vi "PCAN_ERROR_Description.vi"(3 "error":T1 items=["CAN_ERR_OK"=0, "CAN_ERR_XMTFULL"=1, "CAN_ERR_OVERRUN"=2, "CAN_ERR_BUSLIGHT"=4, "CAN_ERR_BUSHEAVY"=8, "CAN_ERR_BUSOFF"=16, "CAN_ERR_QRCVEMPTY"=32, "CAN_ERR_QOVERRUN"=64, "CAN_ERR_QXMTFULL"=128, "CAN_ERR_REGTEST"=256, "CAN_ERR_NOVXD"=512, "CAN_ERR_HWINUSE"=1024, "CAN_ERR_NETINUSE"=2048, "CAN_ERR_ILLHW"=5120, "CAN_ERR_ILLNET"=6144, "CAN_ERR_ILLCLINET"=7168, "CAN_ERR_RESOURCE"=8192, "CAN_ERR_ILLPARAMTYPE"=16384, "CAN_ERR_ILLPARAMVAL"=32768, "CAN_ERR_UNKNOWN"=65536]) -> (1 "Error Description":string)   [LabVIEW 2010]
uses:
  PCAN_ERROR.ctl
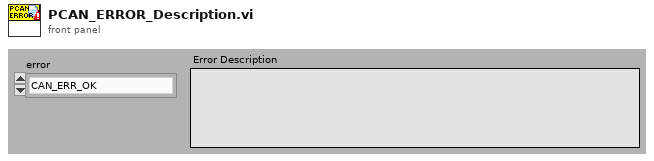
[diagram p1: front panel]
types:
  T1 = typedef "PCAN_ERROR.ctl" = i32
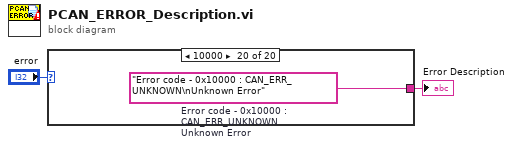
[diagram p0: block diagram]
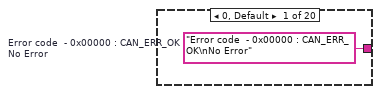
[diagram p2: hidden frame]
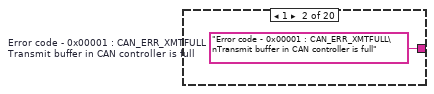
[diagram p3: hidden frame]
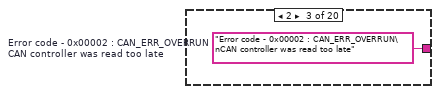
[diagram p4: hidden frame]
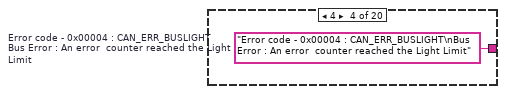
[diagram p5: hidden frame]
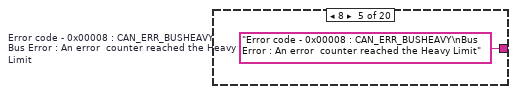
[diagram p6: hidden frame]
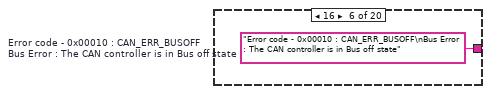
[diagram p7: hidden frame]
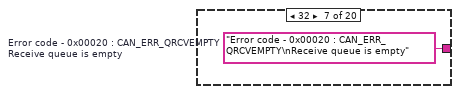
[diagram p8: hidden frame]
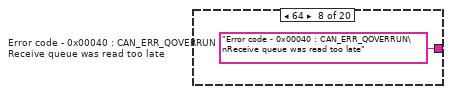
[diagram p9: hidden frame]
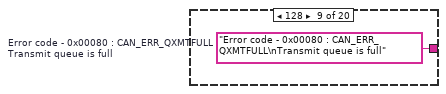
[diagram p10: hidden frame]
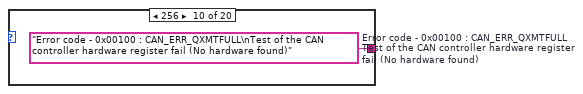
[diagram p11: hidden frame]
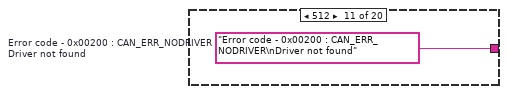
[diagram p12: hidden frame]
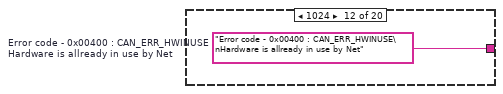
[diagram p13: hidden frame]
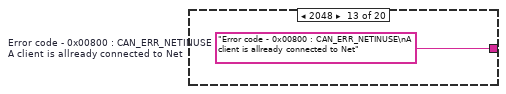
[diagram p14: hidden frame]
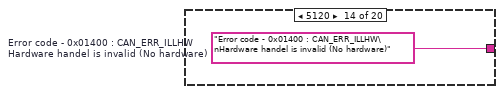
[diagram p15: hidden frame]
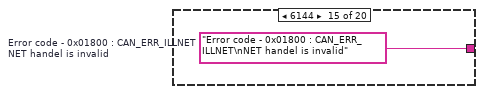
[diagram p16: hidden frame]
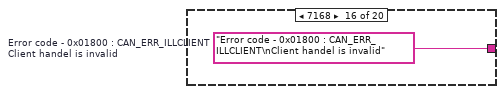
[diagram p17: hidden frame]
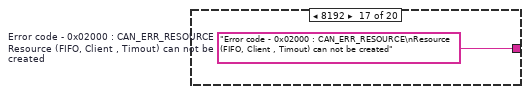
[diagram p18: hidden frame]
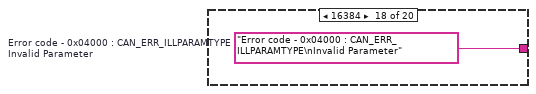
[diagram p19: hidden frame]
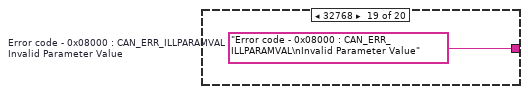
[diagram p20: hidden frame]
diagram:
  n1 = case shown="10000" "error" {
    tunnel: [w3 w4 w5 w6 w7 w8 w9 w10 w11 w12 w13 w14 w15 w16 w17 w18 w19 w20 w21 w22] -> w1
    frame 0, Default {
      w3 = "Error code  - 0x00000 : CAN_ERR_OK\nNo Error"  # Error code  - 0x00000 : CAN_ERR_OK No Error
    }
    frame 1 {
      w4 = "Error code - 0x00001 : CAN_ERR_XMTFULL\nTransmit buffer in CAN controller is full"  # Error code - 0x00001 : CAN_ERR_XMTFULL Transmit buffer in CAN controller is full
    }
    frame 2 {
      w5 = "Error code - 0x00002 : CAN_ERR_OVERRUN\nCAN controller was read too late"  # Error code - 0x00002 : CAN_ERR_OVERRUN CAN controller was read too late
    }
    frame 4 {
      w6 = "Error code - 0x00004 : CAN_ERR_BUSLIGHT\nBus Error : An error  counter reached the Light Limit"  # Error code - 0x00004 : CAN_ERR_BUSLIGHT Bus Error : An error  counter reached the Light Limit
    }
    frame 8 {
      w7 = "Error code - 0x00008 : CAN_ERR_BUSHEAVY\nBus Error : An error  counter reached the Heavy Limit"  # Error code - 0x00008 : CAN_ERR_BUSHEAVY Bus Error : An error  counter reached the Heavy Limit
    }
    frame 16 {
      w8 = "Error code - 0x00010 : CAN_ERR_BUSOFF\nBus Error : The CAN controller is in Bus off state"  # Error code - 0x00010 : CAN_ERR_BUSOFF Bus Error : The CAN controller is in Bus off state
    }
    frame 32 {
      w9 = "Error code - 0x00020 : CAN_ERR_QRCVEMPTY\nReceive queue is empty"  # Error code - 0x00020 : CAN_ERR_QRCVEMPTY Receive queue is empty
    }
    frame 64 {
      w10 = "Error code - 0x00040 : CAN_ERR_QOVERRUN\nReceive queue was read too late"  # Error code - 0x00040 : CAN_ERR_QOVERRUN Receive queue was read too late
    }
    frame 128 {
      w11 = "Error code - 0x00080 : CAN_ERR_QXMTFULL\nTransmit queue is full"  # Error code - 0x00080 : CAN_ERR_QXMTFULL Transmit queue is full
    }
    frame 256 {
      w12 = "Error code - 0x00100 : CAN_ERR_QXMTFULL\nTest of the CAN controller hardware register fail (No hardware found)"  # Error code - 0x00100 : CAN_ERR_QXMTFULL Test of the CAN controller hardware register fail (No hardware found)
    }
    frame 512 {
      w13 = "Error code - 0x00200 : CAN_ERR_NODRIVER\nDriver not found"  # Error code - 0x00200 : CAN_ERR_NODRIVER Driver not found
    }
    frame 1024 {
      w14 = "Error code - 0x00400 : CAN_ERR_HWINUSE\nHardware is allready in use by Net"  # Error code - 0x00400 : CAN_ERR_HWINUSE Hardware is allready in use by Net
    }
    frame 2048 {
      w15 = "Error code - 0x00800 : CAN_ERR_NETINUSE\nA client is allready connected to Net"  # Error code - 0x00800 : CAN_ERR_NETINUSE A client is allready connected to Net
    }
    frame 5120 {
      w16 = "Error code - 0x01400 : CAN_ERR_ILLHW\nHardware handel is invalid (No hardware)"  # Error code - 0x01400 : CAN_ERR_ILLHW Hardware handel is invalid (No hardware)
    }
    frame 6144 {
      w17 = "Error code - 0x01800 : CAN_ERR_ILLNET\nNET handel is invalid"  # Error code - 0x01800 : CAN_ERR_ILLNET NET handel is invalid
    }
    frame 7168 {
      w18 = "Error code - 0x01800 : CAN_ERR_ILLCLIENT\nClient handel is invalid"  # Error code - 0x01800 : CAN_ERR_ILLCLIENT Client handel is invalid
    }
    frame 8192 {
      w19 = "Error code - 0x02000 : CAN_ERR_RESOURCE\nResource (FIFO, Client , Timout) can not be created"  # Error code - 0x02000 : CAN_ERR_RESOURCE Resource (FIFO, Client , Timout) can not be created
    }
    frame 16384 {
      w20 = "Error code - 0x04000 : CAN_ERR_ILLPARAMTYPE\nInvalid Parameter"  # Error code - 0x04000 : CAN_ERR_ILLPARAMTYPE Invalid Parameter
    }
    frame 32768 {
      w21 = "Error code - 0x08000 : CAN_ERR_ILLPARAMVAL\nInvalid Parameter Value"  # Error code - 0x08000 : CAN_ERR_ILLPARAMVAL Invalid Parameter Value
    }
    frame 65536 {
      w22 = "Error code - 0x10000 : CAN_ERR_UNKNOWN\nUnknown Error"  # Error code - 0x10000 : CAN_ERR_UNKNOWN Unknown Error
    }
  }
  "Error Description" <- w1
